vi "Fire Control.vi"() -> ()   [LabVIEW 2011]
panel:
  out "Fire Control":bool
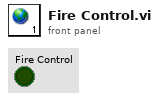
[diagram p1: front panel]
diagram:
